vi "Arrow Drawing Utility.vi"(0 "LF Pod Setpoint":cluster{"Velocity":dbl, "Theta":dbl}, 5 "LB Pod Setpoint":cluster{"Velocity":dbl, "Theta":dbl}, 7 "RF Pod Setpoint":cluster{"Velocity":dbl, "Theta":dbl}, 9 "RB Pod Setpoint":cluster{"Velocity":dbl, "Theta":dbl}, 12 "cross products":T1, 13 "Translation":dbl[](array[numeric])) -> (4 "Pod Vectors":cluster{dbl[], dbl[]}[](array[cluster]), 6 "Translation Vectors":cluster{dbl[], dbl[]}, 8 "Rotation Vectors":cluster{dbl[], dbl[]})   [LabVIEW 2025]
uses:
  <vilib>/ptbypt/NI_PtbyPt.lvlib
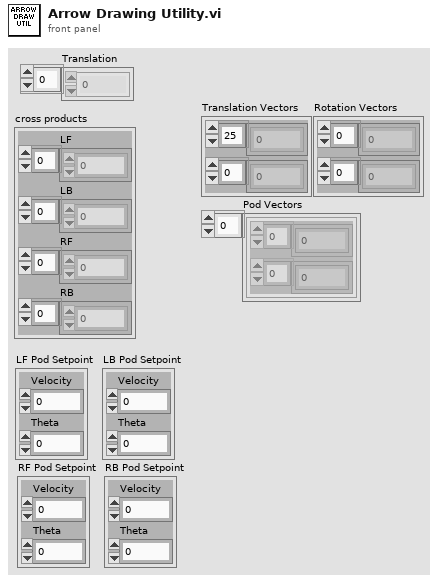
[diagram p1: front panel]
types:
  T1 = cluster{"LF":dbl[], "LB":dbl[], "RF":dbl[], "RB":dbl[]}
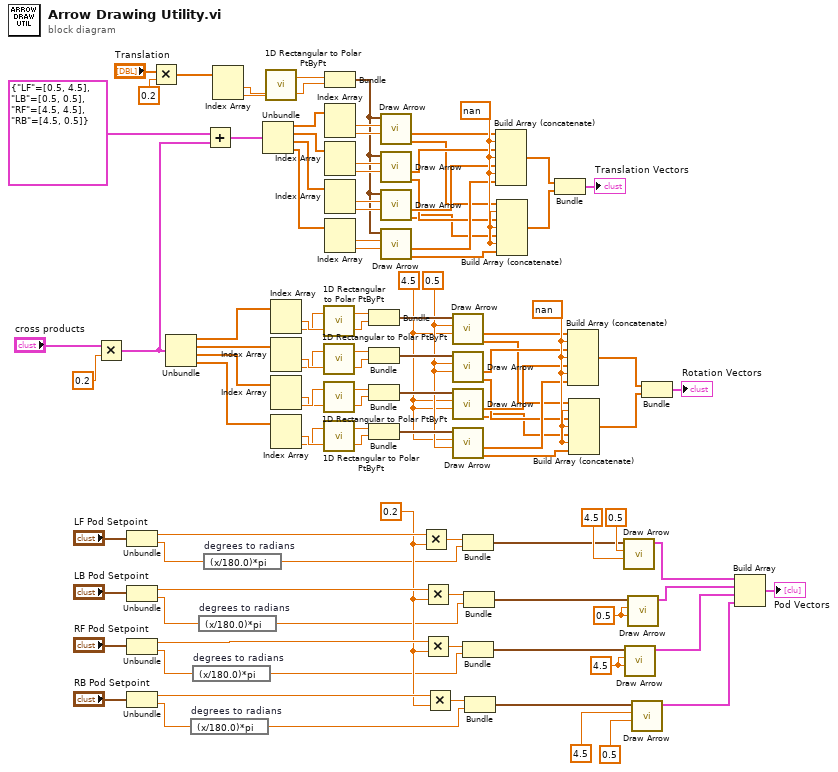
[diagram p0: block diagram]
diagram:
  w49 = nan ("Start Y")
  w62 = nan ("Start Y")
  w63 = 4.5 ("Start Y")
  w64 = 0.5 ("Start X")
  w89 = 0.2 ("y")
  w110 = 4.5 ("Start X")
  w111 = 0.5 ("Start X")
  n1 = Multiply(x="cross products", y=0.2) -> (x*y=w15:T1)
  n2 = Unbundle("LF Pod Setpoint") -> ("Velocity"=w101:dbl, "Theta"=w8:dbl)
  n3 = Unbundle("LB Pod Setpoint") -> ("Velocity"=w100:dbl, "Theta"=w6:dbl)
  n4 = Unbundle("RF Pod Setpoint") -> ("Velocity"=w99:dbl, "Theta"=w4:dbl)
  n5 = Unbundle("RB Pod Setpoint") -> ("Velocity"=w98:dbl, "Theta"=w2:dbl)
  n6 = Multiply(x="Translation", y=0.2) -> (x*y=w17:dbl[])
  n7 = Unbundle(w15) -> ("LF"=w88:dbl[], "LB"=w87:dbl[], "RF"=w86:dbl[], "RB"=w85:dbl[])
  n8 = expression code="(x/180.0)*pi" "degrees to radians"(w2) -> (w1:dbl)
  n9 = expression code="(x/180.0)*pi" "degrees to radians"(w4) -> (w3:dbl)
  n10 = expression code="(x/180.0)*pi" "degrees to radians"(w6) -> (w5:dbl)
  n11 = expression code="(x/180.0)*pi" "degrees to radians"(w8) -> (w7:dbl)
  n12 = Add(x=T1 {"LF"=[0.5, 4.5], "LB"=[0.5, 0.5], "RF"=[4.5, 4.5], "RB"=[4.5, 0.5]}, y=w15) -> (x+y=w50:T1)
  n13 = Index Array(array=w17) -> (element #1=w52:dbl, element #2=w51:dbl)  [unwired: 2 in]
  n14 = Unbundle(w50) -> ("LF"=w40:dbl[], "LB"=w39:dbl[], "RF"=w38:dbl[], "RB"=w37:dbl[])
  n15 = call <vilib>:"1D Rectangular to Polar PtByPt.vi"("y"=w52, "x"=w51) -> ("phase"=w27:dbl, "magnitude"=w28:dbl)
  n16 = Index Array(array=w88) -> (element #1=w84:dbl, element #2=w83:dbl)  [unwired: 2 in]
  n17 = Index Array(array=w87) -> (element #1=w82:dbl, element #2=w78:dbl)  [unwired: 2 in]
  n18 = Index Array(array=w86) -> (element #1=w79:dbl, element #2=w80:dbl)  [unwired: 2 in]
  n19 = Index Array(array=w85) -> (element #1=w81:dbl, element #2=w77:dbl)  [unwired: 2 in]
  n20 = call <vilib>:"1D Rectangular to Polar PtByPt.vi"("y"=w84, "x"=w83) -> ("phase"=w76:dbl, "magnitude"=w75:dbl)
  n21 = call <vilib>:"1D Rectangular to Polar PtByPt.vi"("y"=w82, "x"=w78) -> ("phase"=w71:dbl, "magnitude"=w72:dbl)
  n22 = call <vilib>:"1D Rectangular to Polar PtByPt.vi"("y"=w79, "x"=w80) -> ("phase"=w69:dbl, "magnitude"=w70:dbl)
  n23 = call <vilib>:"1D Rectangular to Polar PtByPt.vi"("y"=w81, "x"=w77) -> ("phase"=w65:dbl, "magnitude"=w66:dbl)
  n24 = Bundle("magnitude"=w28, "phase"=w27) -> (w26:cluster{"magnitude":dbl, "phase":dbl})  [unwired: 1 in]
  n25 = Index Array(array=w40) -> (element #1=w36:dbl, element #2=w35:dbl)  [unwired: 2 in]
  n26 = Index Array(array=w39) -> (element #1=w34:dbl, element #2=w33:dbl)  [unwired: 2 in]
  n27 = Index Array(array=w38) -> (element #1=w32:dbl, element #2=w31:dbl)  [unwired: 2 in]
  n28 = Index Array(array=w37) -> (element #1=w30:dbl, element #2=w29:dbl)  [unwired: 2 in]
  n29 = Bundle("magnitude"=w75, "phase"=w76) -> (w74:cluster{"magnitude":dbl, "phase":dbl})  [unwired: 1 in]
  n30 = Bundle("magnitude"=w72, "phase"=w71) -> (w73:cluster{"magnitude":dbl, "phase":dbl})  [unwired: 1 in]
  n31 = Bundle("magnitude"=w70, "phase"=w69) -> (w68:cluster{"magnitude":dbl, "phase":dbl})  [unwired: 1 in]
  n32 = Bundle("magnitude"=w66, "phase"=w65) -> (w67:cluster{"magnitude":dbl, "phase":dbl})  [unwired: 1 in]
  n33 = call "Draw Arrow.vi"("Start Y"=w35, "Start X"=w36, "Vector"=w26) -> ("Y"=w44:dbl[], "X"=w48:dbl[])  [unwired: 6 in, 1 out]
  n34 = call "Draw Arrow.vi"("Start Y"=w33, "Start X"=w34, "Vector"=w26) -> ("Y"=w43:dbl[], "X"=w47:dbl[])  [unwired: 6 in, 1 out]
  n35 = call "Draw Arrow.vi"("Start Y"=w31, "Start X"=w32, "Vector"=w26) -> ("Y"=w42:dbl[], "X"=w46:dbl[])  [unwired: 6 in, 1 out]
  n36 = call "Draw Arrow.vi"("Start Y"=w29, "Start X"=w30, "Vector"=w26) -> ("Y"=w41:dbl[], "X"=w45:dbl[])  [unwired: 6 in, 1 out]
  n37 = Multiply(x=w101, y=w89) -> (x*y=w97:dbl)
  n38 = Multiply(x=w100, y=w89) -> (x*y=w94:dbl)
  n39 = Multiply(x=w99, y=w89) -> (x*y=w96:dbl)
  n40 = Multiply(x=w98, y=w89) -> (x*y=w95:dbl)
  n41 = call "Draw Arrow.vi"("Start Y"=w63, "Start X"=w64, "Vector"=w74) -> ("Y"=w57:dbl[], "X"=w61:dbl[])  [unwired: 6 in, 1 out]
  n42 = call "Draw Arrow.vi"("Start Y"=w64, "Start X"=w64, "Vector"=w73) -> ("Y"=w56:dbl[], "X"=w60:dbl[])  [unwired: 6 in, 1 out]
  n43 = call "Draw Arrow.vi"("Start Y"=w63, "Start X"=w63, "Vector"=w68) -> ("Y"=w55:dbl[], "X"=w59:dbl[])  [unwired: 6 in, 1 out]
  n44 = call "Draw Arrow.vi"("Start Y"=w64, "Start X"=w63, "Vector"=w67) -> ("Y"=w54:dbl[], "X"=w58:dbl[])  [unwired: 6 in, 1 out]
  n45 = Bundle(w97, "Theta"=w7) -> (w93:cluster{dbl, "Theta":dbl})  [unwired: 1 in]
  n46 = Bundle(w96, "Theta"=w3) -> (w91:cluster{dbl, "Theta":dbl})  [unwired: 1 in]
  n47 = Bundle(w94, "Theta"=w5) -> (w92:cluster{dbl, "Theta":dbl})  [unwired: 1 in]
  n48 = Bundle(w95, "Theta"=w1) -> (w90:cluster{dbl, "Theta":dbl})  [unwired: 1 in]
  n49 = Build Array (concatenate)(w48, w49, w47, w49, w46, w49, w45) -> (w25:dbl[])
  n50 = Build Array (concatenate)(w44, w49, w43, w49, w42, w49, w41) -> (w24:dbl[])
  n51 = Bundle(w25, w24) -> (→"Translation Vectors":cluster{dbl[], dbl[]})  [unwired: 1 in]
  n52 = Build Array (concatenate)(w61, w62, w60, w62, w59, w62, w58) -> (w23:dbl[])
  n53 = Build Array (concatenate)(w57, w62, w56, w62, w55, w62, w54) -> (w22:dbl[])
  n54 = call "Draw Arrow.vi"("Start Y"=4.5, "Start X"=0.5, "Vector"=w93) -> ("Points"=w13:cluster{dbl[], dbl[]})  [unwired: 6 in, 2 out]
  n55 = call "Draw Arrow.vi"("Start Y"=w110, "Start X"=w110, "Vector"=w91) -> ("Points"=w11:cluster{dbl[], dbl[]})  [unwired: 6 in, 2 out]
  n56 = call "Draw Arrow.vi"("Start Y"=w111, "Start X"=w111, "Vector"=w92) -> ("Points"=w12:cluster{dbl[], dbl[]})  [unwired: 6 in, 2 out]
  n57 = call "Draw Arrow.vi"("Start Y"=0.5, "Start X"=4.5, "Vector"=w90) -> ("Points"=w10:cluster{dbl[], dbl[]})  [unwired: 6 in, 2 out]
  n58 = Bundle(w23, w22) -> (→"Rotation Vectors":cluster{dbl[], dbl[]})  [unwired: 1 in]
  n59 = Build Array(w13, w12, w11, w10) -> (→"Pod Vectors":cluster{dbl[], dbl[]}[])
